vi "registered.vi"() -> ()   [LabVIEW 2013]
uses:
  IOTFoundation.lvlib
panel:
  in  "Message to transmit":string="{\"foo\": \"bar\"}"
  in  "Device name":string="default"
  in  "Credentials file path":path=path "c:/ni-rt/config/iotf-credentials.ini"
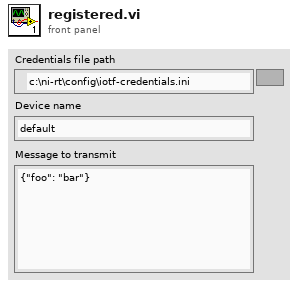
[diagram p1: front panel]
types:
  T1 = cluster{"Organization":string, "Device Type":string, "Device ID":string, "Auth token":string}
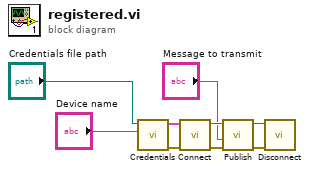
[diagram p0: block diagram]
diagram:
  n1 = call "Credentials.vi"("Path"="Credentials file path", "Device Name"="Device name") -> ("Cluster"=w9:T1, "error out"=w8:errorcluster)  [unwired: 6 in, 1 out]
  n2 = call "Connect.vi"("Credentials"=w9, "error in (no error)"=w8) -> ("connection ID out"=w7:refnum<k5>, "error out"=w6:errorcluster)  [unwired: 5 in, 1 out]
  n3 = call "Publish.vi"("error in (no error)"=w6, "Message to be published"="Message to transmit", "connection ID"=w7) -> ("error out"=w4:errorcluster, "connection ID out"=w5:refnum<k5>)  [unwired: 7 in]
  n4 = call "Disconnect.vi"("error in (no error)"=w4, "connection ID"=w5) -> ()  [unwired: 9 in, 1 out]
